vi "Read Connected Camera.vi"(8 "error in (no error)":errorcluster, 11 "Realsense Cam in":refnum<class "Realsense Cam.lvclass">) -> (0 "error out":errorcluster, 2 "Connected Camera":T1, 3 "Realsense Cam out":refnum<class "Realsense Cam.lvclass">)   [LabVIEW 2018, in "Realsense Cam.lvclass"]
uses:
  Realsense Cam.lvclass
  Private/Camera Connection STYP.ctl
  Realsense Cam.lvclass/Realsense Cam.ctl
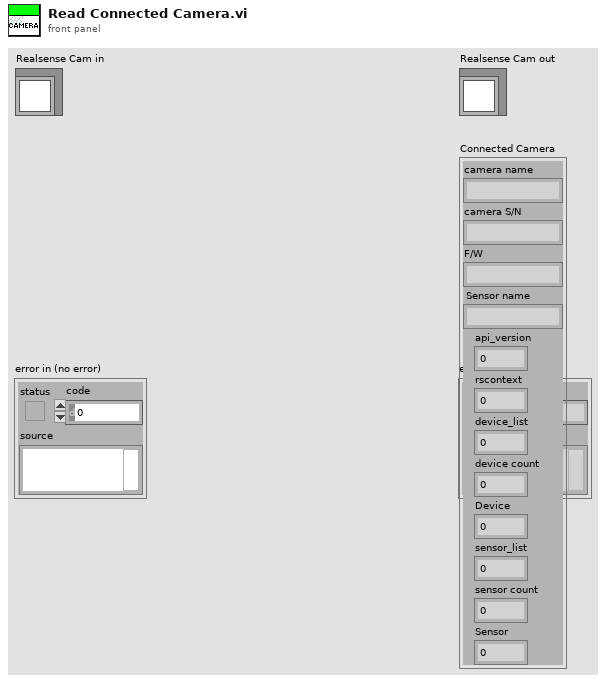
[diagram p1: front panel]
types:
  T1 = typedef "Realsense Cam.lvclass/Camera Connection STYP.ctl" = cluster{"camera name":string, "camera S/N":string, "F/W":string, "Sensor name":string, "api_version":i32, "rscontext":u64, "device_list":u64, "device count":i32, "Device":u64, "sensor_list":u64, "sensor count":i32, "Sensor":u64}
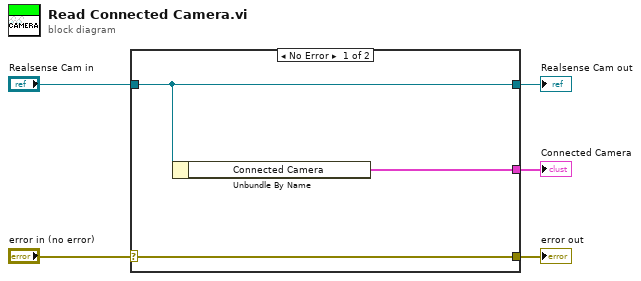
[diagram p0: block diagram]
diagram:
  n1 = case shown="No Error" "error in (no error)" {
    selector: "error in (no error)" -> [w8 w9]
    tunnel: [w8 w9] -> w4
    tunnel: [w7 w10] -> w2
    tunnel: "Realsense Cam in" -> [w7 w10]
    tunnel: [w6 _] -> w1
    frame No Error {
      n2 = Unbundle By Name(w7) -> ("Connected Camera"=w6:T1)
    }
    frame Error {
    }
  }
  "error out" <- w4
  "Realsense Cam out" <- w2
  "Connected Camera" <- w1
